vi "Building_Variants_after_Origin(11)-2.vi"(4 "[IN] Minimal Subtrack Length":i32, 5 "[IN] Subtrack":T1, 6 "[IN] Index in the Subtrack":i32, 7 "[IN] Indexes for Jumps":i32[](array[numeric]), 8 "error IN":errorcluster, 9 "[IN] Count of variants":i32, 10 "[IN] Subtracks":T3(array[cluster]), 11 "[IN] Still connected\ntracks in group":T2) -> (0 "error OUT":errorcluster, 1 "[OUT] Count of variants":i32, 2 "[OUT] Subtracks":T3(array[cluster]))   [LabVIEW 2013]
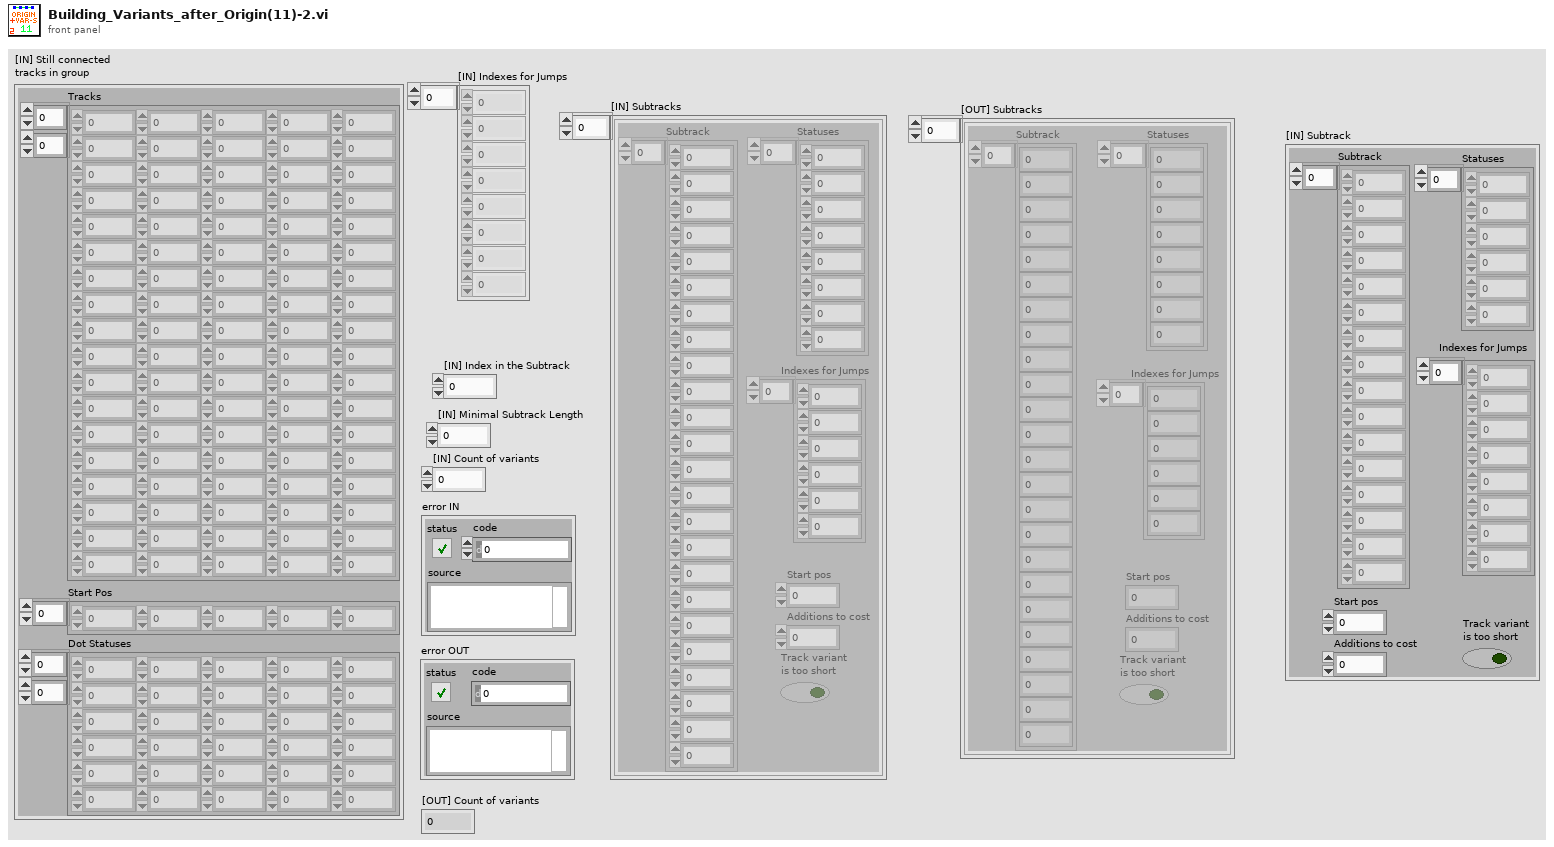
[diagram p1: front panel]
types:
  T1 = cluster{"Subtrack":dbl[], "Statuses":i16[], "Start pos":i32, "Additions to cost":i32, "Track variant \nis too short":bool, "Indexes for Jumps":i32[]}
  T2 = cluster{"Tracks":dbl[][], "Start Pos":i32[], "Dot Statuses":i16[][]}
  T3 = cluster{"Subtrack":dbl[], "Statuses":i16[], "Start pos":i32, "Additions to cost":i32, "Track variant \nis too short":bool, "Indexes for Jumps":i32[]}[]
  T4 = cluster{"Subtrack":dbl[], "Statuses":i16[], "Start pos":i32, "Additions to cost":i8, "Track variant \nis too short":bool, "Indexes for Jumps":i32[]}
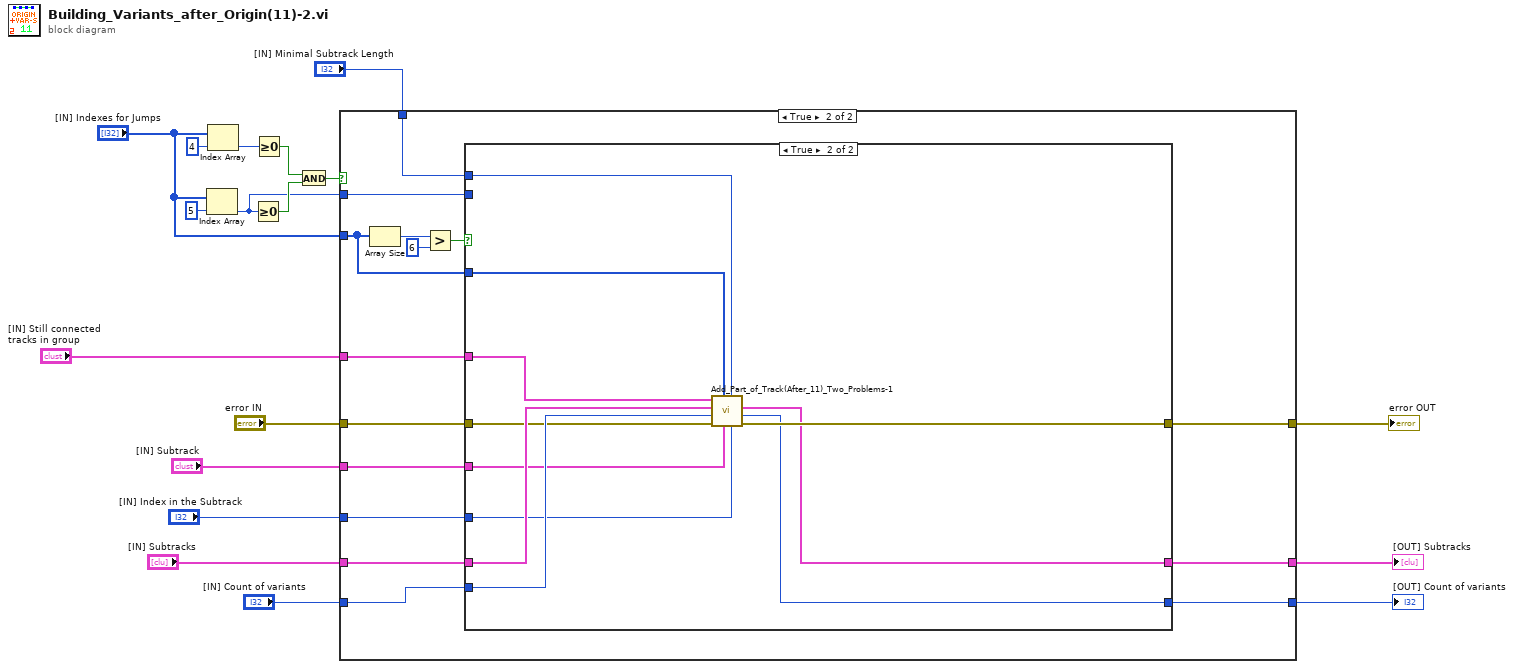
[diagram p0: block diagram]
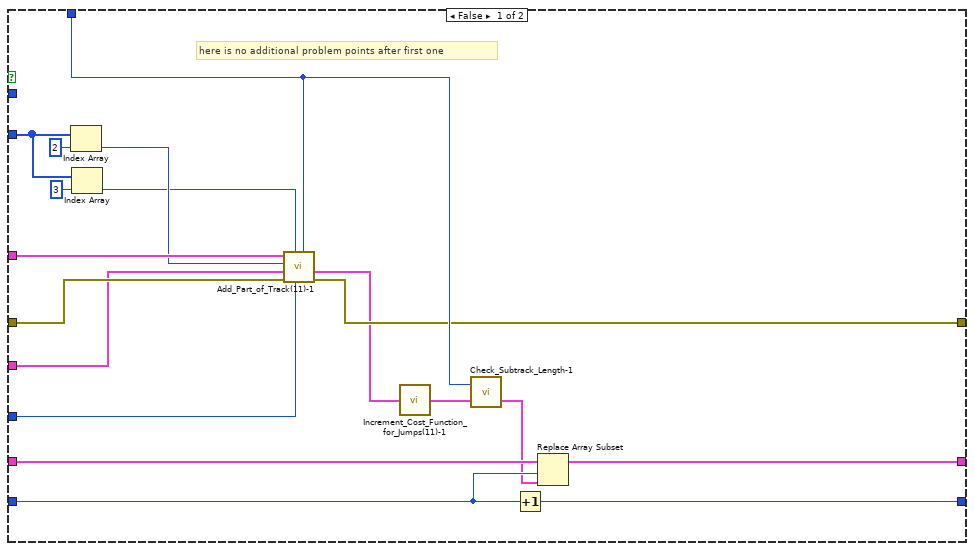
[diagram p2: hidden frame]
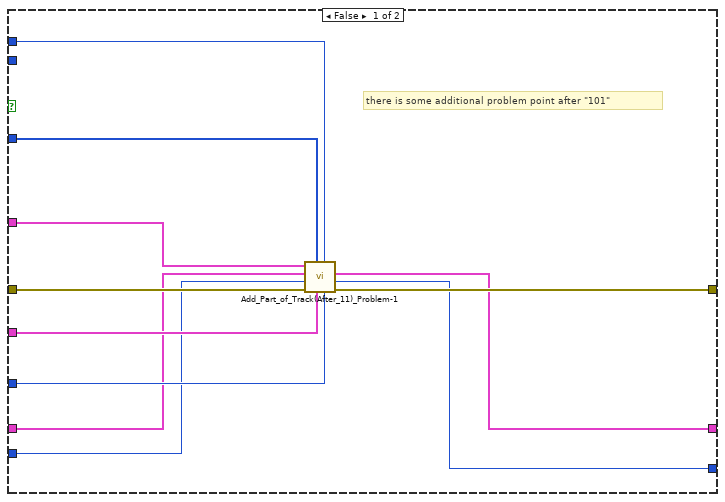
[diagram p3: hidden frame]
diagram:
  n1 = Index Array(array="[IN] Indexes for Jumps", index=5) -> (element=w12:i32)
  n2 = Index Array(array="[IN] Indexes for Jumps", index=4) -> (element=w13:i32)
  n3 = Greater Or Equal To 0?(x=w12) -> (x >= 0?=w15:bool)
  n4 = Greater Or Equal To 0?(x=w13) -> (x >= 0?=w16:bool)
  n5 = And(x=w16, y=w15) -> (x .and. y?=w14:bool)
  n6 = case shown="True" w14 {
    tunnel: w12 -> [_ w47]
    tunnel: "[IN] Indexes for Jumps" -> [w34 w40]
    tunnel: "[IN] Still connected\ntracks in group" -> [w30 w46]
    tunnel: "[IN] Subtrack" -> [w26 w48]
    tunnel: "error IN" -> [w29 w45]
    tunnel: "[IN] Index in the Subtrack" -> [w27 w43]
    tunnel: "[IN] Minimal Subtrack Length" -> [w28 w44]
    tunnel: "[IN] Subtracks" -> [w33 w42]
    tunnel: "[IN] Count of variants" -> [w32 w41]
    tunnel: [w23 w39] -> w1
    tunnel: [w22 w38] -> w2
    tunnel: [w21 w37] -> w3
    frame False {
      # "here is no additional problem points after first one"
      n7 = Index Array(array=w34, index=2) -> (element=w25:i32)
      n8 = Index Array(array=w34, index=3) -> (element=w24:i32)
      n9 = call "Add_Part_of_Track(11)-1.vi"("[IN] Minimal Sub\ntrack Length"=w28, "[IN] Index in subtrack"=w27, "[IN] # of subtrack conta\nining problem point"=w24, "error IN"=w29, "[IN] Subtrack"=w26, "[IN] Index of problem\npoint inside subtrack"=w25, "[IN] Still connected\ntracks in group"=w30) -> ("error OUT"=w21:errorcluster, "[OUT] Subtrack"=w20:T1)  [unwired: 2 in, 1 out]
      n10 = call "Increment_Cost_Function_for_Jumps(11)-1.vi"("[IN] Subtrack"=w20) -> ("[OUT] Subtrack"=w19:T1)
      n11 = call "Check_Subtrack_Length-1.vi"("[IN] Subtrack"=w19, "[IN] Minimal Sub\ntrack Length"=w28) -> ("[OUT] Subtrack"=w31:T4)  [unwired: 1 in]
      n12 = Increment(x=w32) -> (x+1=w22:i32)
      n13 = Replace Array Subset(array=w33, new element=w31, index=w32) -> (w23:T3)
    }
    frame True {
      n14 = Array Size(array=w40) -> (size(s)=w51:i32)
      n15 = Greater?(x=w51, y=6) -> (0:w49:bool)
      n16 = case shown="True" w49 {
        tunnel: w48 -> [w60 w66]
        tunnel: w47 -> [_ _]
        tunnel: w46 -> [w56 w73]
        tunnel: w45 -> [w62 w70]
        tunnel: w44 -> [w54 w67]
        tunnel: w43 -> [w59 w65]
        tunnel: w42 -> [w58 w72]
        tunnel: w41 -> [w57 w71]
        tunnel: [w53 w64] -> w39
        tunnel: [w52 w63] -> w38
        tunnel: w40 -> [w55 w68]
        tunnel: [w61 w69] -> w37
        frame False {
          # "there is some additional problem point after \"101\""
          n17 = call "Add_Part_of_Track(After_11)_Problem-1.vi"("[IN] Index in subtrack"=w59, "[IN] Minimal Sub\ntrack Length"=w54, "[IN] Subtrack"=w60, "[IN] Indexes for Jumps"=w55, "error IN"=w62, "[IN] Count of variants"=w57, "[IN] Subtracks"=w58, "[IN] Still connected\ntracks in group"=w56) -> ("error OUT"=w61:errorcluster, "[OUT] Count of variants"=w52:i32, "[OUT] Subtracks"=w53:T3)  [unwired: 1 in]
        }
        frame True {
          n18 = call "Add_Part_of_Track(After_11)_Two_Problems-1.vi"("[IN] Index in subtrack"=w65, "[IN] Minimal Sub\ntrack Length"=w67, "[IN] Subtrack"=w66, "[IN] Indexes for Jumps"=w68, "error IN"=w70, "[IN] Count of variants"=w71, "[IN] Subtracks"=w72, "[IN] Still connected\ntracks in group"=w73) -> ("error OUT"=w69:errorcluster, "[OUT] Count of variants"=w63:i32, "[OUT] Subtracks"=w64:T3)  [unwired: 1 in]
        }
      }
    }
  }
  "[OUT] Subtracks" <- w1
  "error OUT" <- w3
  "[OUT] Count of variants" <- w2
